vi "ROI from INI Section.vi"(8 "error in (no error)":errorcluster, 11 "refnum in":T1) -> (0 "error out":errorcluster, 2 "ROI":T2 {"Contours"."Type" items=["No Selection", "Point", "Line", "Rectangle", "Oval", "Polygon", "Freehand Region", "Annulus", "Unused2", "Unused3", "Broken Line", "Freehand Line", "Rotated Rectangle"]}, 3 "refnum out":T1)   [LabVIEW 2020]
uses:
  <vilib>/Utility/config.llb/Config Data RefNum.ctl
  <vilib>/Utility/config.llb/Read Key (I32).vi
  <vilib>/Utility/config.llb/NI_LVConfig.lvlib
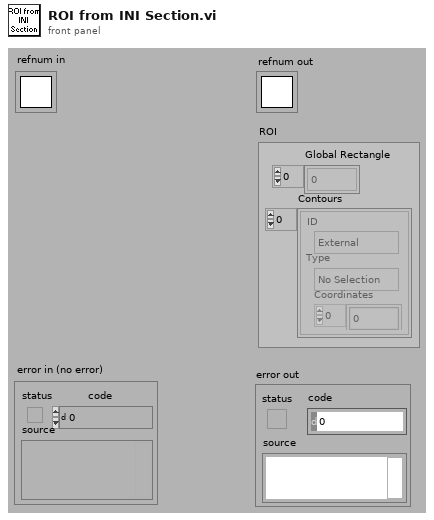
[diagram p1: front panel]
types:
  T1 = typedef "NI_LVConfig.lvlib/Config Data RefNum.ctl" = refnum<k1>
  T2 = typedef "ROI Descriptor" = cluster{"Global Rectangle":i32[], "Contours":cluster{"ID":enum32{"External", "Internal"}, "Type":u32, "Coordinates":i32[]}[]}
  T3 = cluster{"ID":enum32{"External", "Internal"}, "Type":u32, "Coordinates":i32[]}[]
  T4 = cluster{"ID":enum32{"External", "Internal"}, "Type":u32, "Coordinates":i32[]}
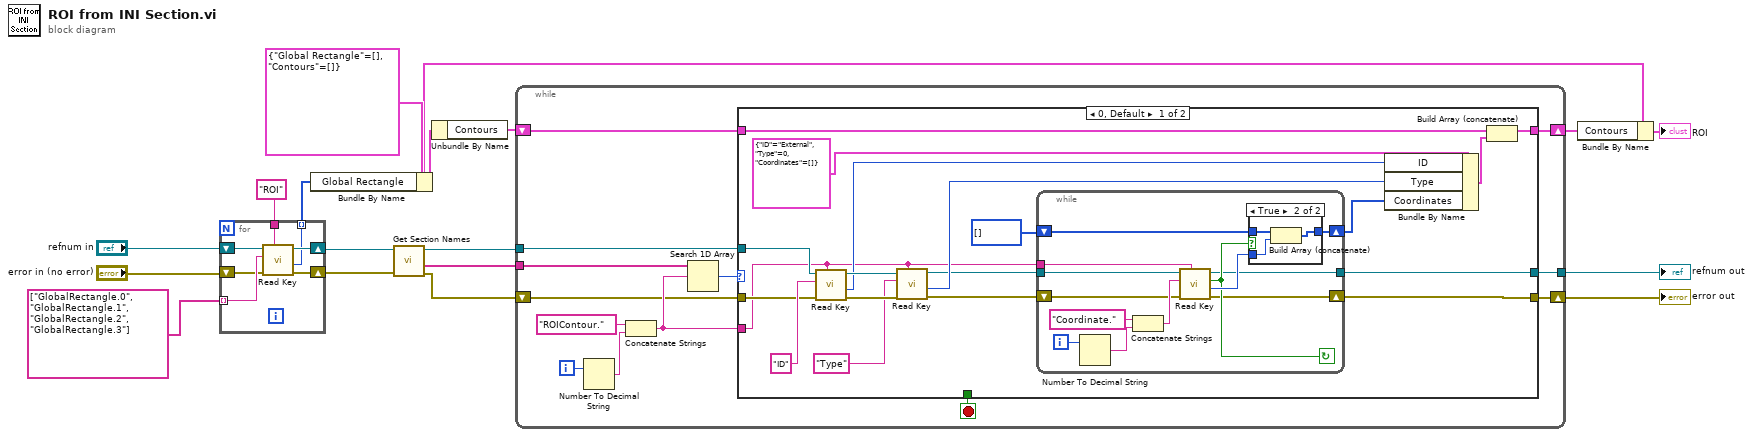
[diagram p0: block diagram]
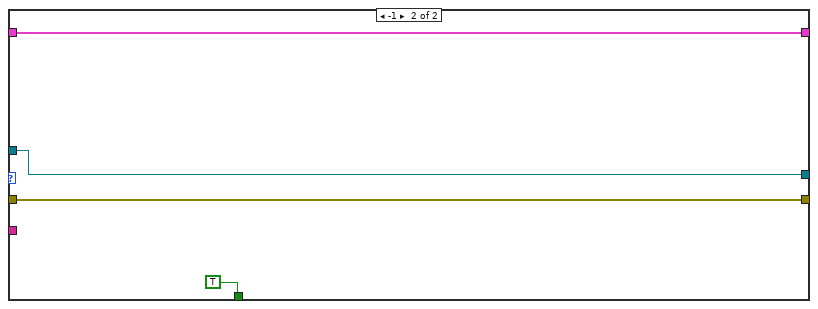
[diagram p3: hidden frame]
diagram:
  n1 = for {
    tunnel: string[] ["GlobalRectangle.0", "GlobalRectangle.1", "GlobalRectangle.2", "GlobalRectangle.3"] -> [w23] mode=indexing
    shift-right: [w22] -> w3
    shift-left: "refnum in" -> [w24]
    shift-right: [w20] -> w4
    shift-left: "error in (no error)" -> [w21]
    tunnel: [w19] -> w11 mode=indexing
    tunnel: "ROI" ("section") -> [w18]
    n2 = call-poly <vilib>:"Read Key.vi"("section"=w18, "error in (no error)"=w21, "key"=w23, "refnum"=w24) -> ("error out"=w20:errorcluster, "value"=w19:i32, "refnum out"=w22:T1)  [unwired: 4 in, 1 out]
  }
  n3 = Bundle By Name(cluster=T2 {"Global Rectangle"=[], "Contours"=[]} ("ROI Descriptor"), "Global Rectangle"=w11) -> (w9:T2)
  n4 = call <vilib>:"Get Section Names.vi"("error in (no error)"=w4, "refnum"=w3) -> ("error out"=w1:errorcluster, "section names"=w10:string[], "refnum out"=w2:T1)  [unwired: 7 in]
  n5 = Unbundle By Name(w9) -> ("Contours"=w15:T3)
  n6 = while {
    tunnel: w10 -> [w37]
    tunnel: w2 -> [w30]
    shift-right: [w28] -> w16
    shift-left: w1 -> [w29]
    tunnel: [w27] -> w17
    shift-right: [w25] -> w8
    shift-left: w15 -> [w26]
    i -> [w34]
    stop <- w32 stop-if-true
    n7 = Number To Decimal String(number=w34) -> (decimal integer string=w36:string)  [unwired: 1 in]
    n8 = Concatenate Strings("ROIContour." ("section"), w36) -> (w31:string)
    n9 = Search 1D Array(1D array=w37, element=w31) -> (index of element=w33:i32)  [unwired: 1 in]
    n10 = case shown="0, Default" w33 {
      tunnel: [_ TRUE] -> w32
      tunnel: w31 -> [w45 _]
      tunnel: w30 -> [w55 w75]
      tunnel: w29 -> [w54 w76]
      tunnel: w26 -> [w39 w74]
      tunnel: [w43 w76] -> w28
      tunnel: [w42 w75] -> w27
      tunnel: [w38 w74] -> w25
      frame 0, Default {
        n11 = call-poly <vilib>:"Read Key.vi"("section"=w45, "error in (no error)"=w54, "key"="ID", "refnum"=w55) -> ("error out"=w53:errorcluster, "value"=w49:i32, "refnum out"=w52:T1)  [unwired: 4 in, 1 out]
        n12 = call-poly <vilib>:"Read Key.vi"("section"=w45, "error in (no error)"=w53, "key"="Type", "refnum"=w52) -> ("error out"=w47:errorcluster, "value"=w48:i32, "refnum out"=w46:T1)  [unwired: 4 in, 1 out]
        n13 = while {
          tunnel: w46 -> [w65]
          tunnel: w45 -> [w66]
          shift-right: [w62] -> w41
          shift-left: i32[] [] ("Coordinates") -> [w64]
          shift-right: [w58] -> w43
          shift-left: w47 -> [w60]
          tunnel: [w57] -> w42
          i -> [w67]
          stop <- w59 continue-if-true
          n14 = Number To Decimal String(number=w67) -> (decimal integer string=w68:string)  [unwired: 1 in]
          n15 = Concatenate Strings("Coordinate." ("string"), w68) -> (w61:string)
          n16 = call-poly <vilib>:"Read Key.vi"("section"=w66, "error in (no error)"=w60, "key"=w61, "refnum"=w65) -> ("error out"=w58:errorcluster, "value"=w63:i32, "found?"=w59:bool, "refnum out"=w57:T1)  [unwired: 4 in]
          n17 = case shown="True" w59 {
            tunnel: w64 -> [w70 w73]
            tunnel: w63 -> [_ w72]
            tunnel: [w70 w71] -> w62
            frame False {
            }
            frame True {
              n18 = Build Array (concatenate)(w73, w72) -> (w71:i32[])
            }
          }
        }
        n19 = Bundle By Name(cluster=T4 {"ID"=enum."External", "Type"=0, "Coordinates"=[]} ("element"), "ID"=w49, "Type"=w48, "Coordinates"=w41) -> (w40:T4)
        n20 = Build Array (concatenate)(w39, w40) -> (w38:T3)
      }
      frame -1 {
      }
    }
  }
  "error out" <- w16
  "refnum out" <- w17
  n21 = Bundle By Name(cluster=w9, "Contours"=w8) -> (→"ROI":T2)
